vi "Unsubscribe (Scalar).vi"(6 "timeout (1000ms)":i32=1000, 8 "error in (no error)":errorcluster, 10 "Topic Filter":string, 11 "Client in":refnum<class "Client.lvclass">) -> (0 "error out":errorcluster, 1 "Ack":bool, 3 "Client out":refnum<class "Client.lvclass">)   [LabVIEW 2013, in "MQTT Client.lvlib" / "Client.lvclass"]
uses:
  Client.lvclass
  <vilib>/LabVIEW Open Source Project/MQTT Connection/MQTT_Base/Base Class/MQTT_Base.lvclass
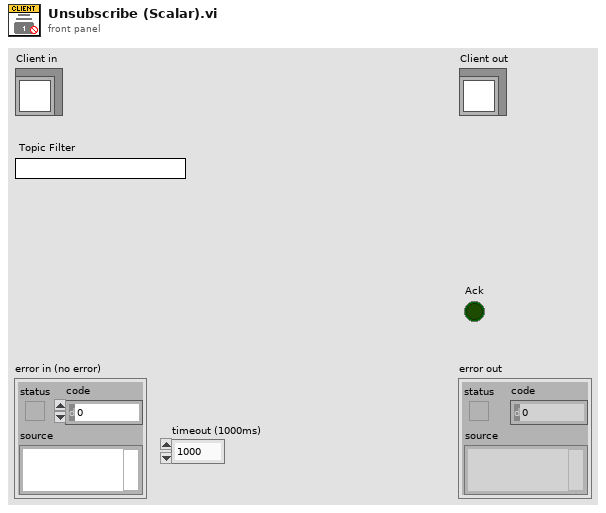
[diagram p1: front panel]
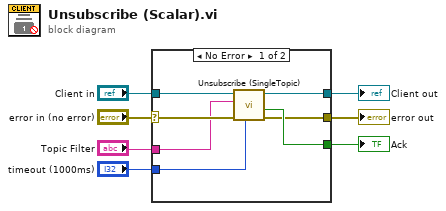
[diagram p0: block diagram]
diagram:
  n1 = case shown="No Error" "error in (no error)" {
    selector: "error in (no error)" -> [w10 w16]
    tunnel: [w11 w16] -> w6
    tunnel: [w13 w15] -> w4
    tunnel: "Client in" -> [w14 w15]
    tunnel: [w12 _] -> w3
    tunnel: "Topic Filter" -> [w9 _]
    tunnel: "timeout (1000ms)" -> [w8 _]
    frame No Error {
      n2 = call <vilib>:"Unsubscribe (SingleTopic).vi"("timeout (100ms)"=w8, "error in (no error)"=w10, "Topic Filter"=w9, "MQTT_Base in"=w14) -> ("error out"=w11:errorcluster, "Ack"=w12:bool, "MQTT_Base out"=w13:refnum<class "Client.lvclass">)  [unwired: 5 in]
    }
    frame Error {
    }
  }
  "error out" <- w6
  "Client out" <- w4
  "Ack" <- w3
